vi "Self-Test.vi"(8 "error in (no error)":errorcluster, 11 "VISA resource name":refnum<visa-resource-name>) -> (0 "error out":errorcluster, 1 "Self-Test Result Message":string, 2 "Self-Test Result Code":i32, 3 "VISA resource name out":refnum<visa-resource-name>)   [LabVIEW 2014, in "YbTempCtrl.lvlib"]
doc: "Runs the instrument's self-test routine and returns the test results."
uses:
  YbTempCtrl.lvlib
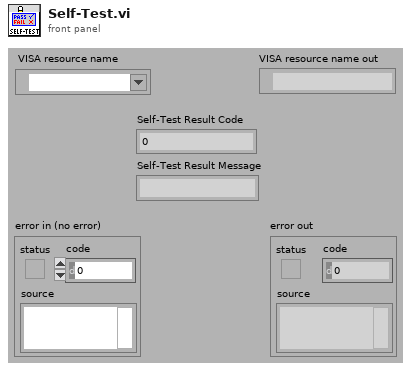
[diagram p1: front panel]
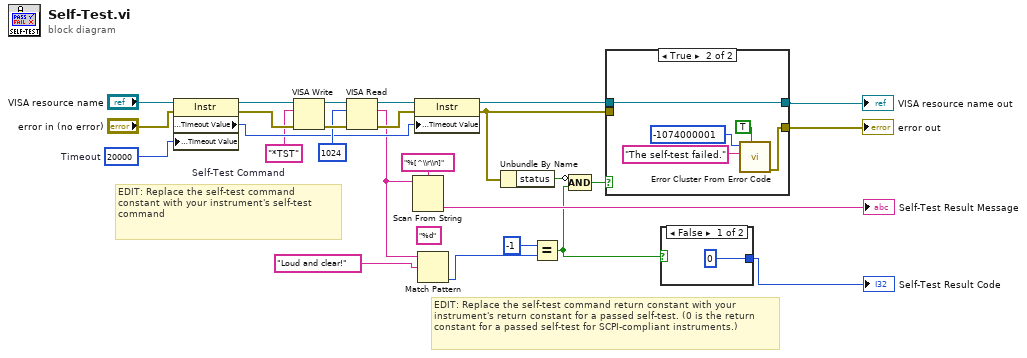
[diagram p0: block diagram]
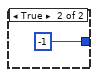
[diagram p2: hidden frame]
diagram:
  w17 = u32 20000  # Timeout
  w13 = "*TST"  # Self-Test Command
  (unwired) "%d" ("format string")
  # "EDIT: Replace the self-test command return constant with your instrument's return constant for a passed self-test. (0 is the return constant for a passed self-test for SCPI-compliant instruments.)"
  # "EDIT: Replace the self-test command constant with your instrument's self-test command"
  n1 = property class="Instr"(reference="VISA resource name", error in="error in (no error)", "General Settings:Timeout Value"=w17) -> (reference out=w15:refnum<visa-resource-name>, error out=w16:errorcluster, "General Settings:Timeout Value"=w14:u32)
  n2 = VISA Write(VISA resource name=w15, write buffer=w13, error in (no error)=w16) -> (VISA resource name out=w23:refnum<visa-resource-name>, error out=w22:errorcluster)  [unwired: 1 out]
  n3 = VISA Read(VISA resource name=w23, byte count=u32 1024 ("byte count (20)"), error in (no error)=w22) -> (VISA resource name out=w25:refnum<visa-resource-name>, read buffer=w6:string, error out=w24:errorcluster)  [unwired: 1 out]
  n4 = Scan From String(format string="%[^\\r\\n]" ("Format String"), input string=w6) -> (output 1=→"Self-Test Result Message":string)  [unwired: 3 in, 3 out]
  n5 = property class="Instr"(reference=w25, error in=w24, "General Settings:Timeout Value"=w14) -> (reference out=w12:refnum<visa-resource-name>, error out=w11:errorcluster)
  n6 = Match Pattern(string=w6, regular expression="Loud and clear!" ("Format String")) -> (offset past match=w4:i32)  [unwired: 1 in, 3 out]
  n7 = Unbundle By Name(w11) -> ("status"=w10:bool)
  n8 = Equal?(x=-1, y=w4) -> (x = y?=w2:bool)
  n9 = Compound Arithmetic op=AND(invert w10, w2) -> (w9:bool)
  n10 = case shown="True" w9 {
    tunnel: w12 -> [w28 w33]
    tunnel: w11 -> [w27 _]
    tunnel: [w27 w29] -> w8
    tunnel: [w28 w33] -> w7
    frame False {
    }
    frame True {
      n11 = call <vilib>:"Error Cluster From Error Code.vi"("show call chain? (False)"=TRUE, "error message (\"\")"="The self-test failed." ("Source (VI Name)"), "error code (0)"=-1074000001 ("Code")) -> ("error out"=w29:errorcluster)  [unwired: 6 in]
    }
  }
  "VISA resource name out" <- w7
  "error out" <- w8
  n12 = case shown="False" w2 {
    tunnel: [0 ("x") -1 ("x")] -> w1
    frame False {
    }
    frame True {
    }
  }
  "Self-Test Result Code" <- w1
